vi "FTW-JSON-Object-DeleteAllElements.vi"(0 "JSON Object":refnum<class "FTW-JSON.lvclass">, 11 "error in":errorcluster) -> (4 "JSON Object out":refnum<class "FTW-JSON.lvclass">, 6 "Success?":bool, 15 "error out":errorcluster)   [LabVIEW 2013, in "FTW-JSON.lvclass"]
uses:
  FTW-JSON.lvclass
  FTW-JSON.lvclass/FTW-JSON.ctl
panel:
  # "Inputs"
  # "Outputs"
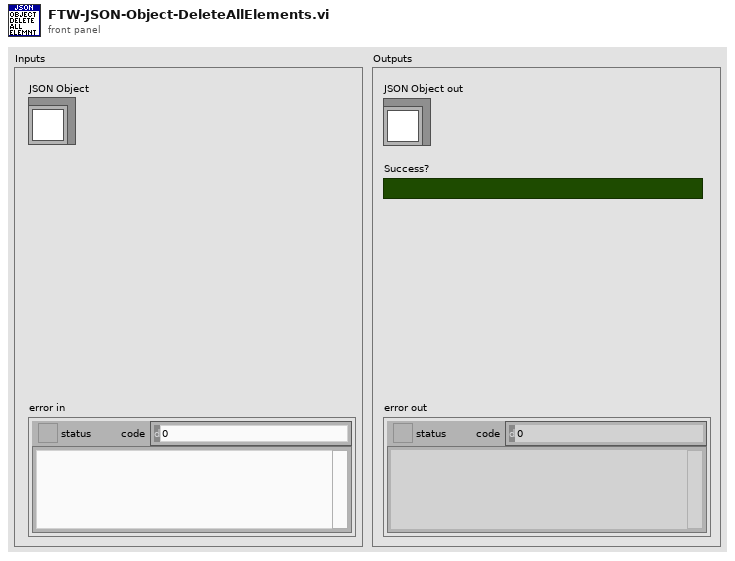
[diagram p1: front panel]
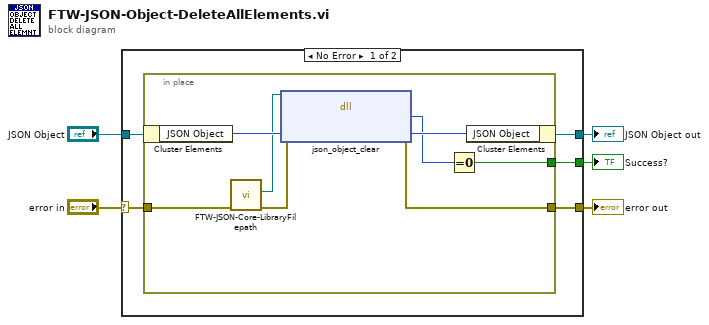
[diagram p0: block diagram]
diagram:
  n1 = case shown="No Error" "error in" {
    selector: "error in" -> [w10 w20]
    tunnel: [w7 w20] -> w5
    tunnel: [w8 w19] -> w3
    tunnel: "JSON Object" -> [w9 w19]
    tunnel: [w6 _] -> w1
    frame No Error {
      n2 = in-place {
        in-place-border: w10 -> [w18]
        in-place-border: [w14] -> w7
        in-place-border: [w11] -> w6
        n3 = in-place-cluster #1(w9) -> ("JSON Object"=w17:i64)
        n4 = call "FTW-JSON-Core-LibraryFilepath.vi"("error in"=w18) -> ("error out"=w16:errorcluster, "JSON Library Filepath"=w15:path)  [unwired: 9 in]
        n5 = dll-call lib="?" fn="json_object_clear"(path in=w15, error in=w16, "JSON Object Pointer"=w17) -> (error out=w14:errorcluster, "Return Value"=w12:i64, "JSON Object Pointer"=w13:i64)  [unwired: 1 in, 1 out]
        n6 = Equal To 0?(x=w12) -> (x = 0?=w11:bool)
        n7 = in-place-cluster #1("JSON Object"=w13) -> (w8:refnum<class "FTW-JSON.lvclass">)
      }
    }
    frame Error {
    }
  }
  "error out" <- w5
  "JSON Object out" <- w3
  "Success?" <- w1
